vi "ROI_to_Size.vi"(11 "Actual ROI":T1 {"Rotation" format="%.2f"; "Left" scale=0.0..1024.0; "Right" scale=0.0..1024.0}) -> (3 "Image Size":cluster{"X":i32, "Y":i32})   [LabVIEW 2014]
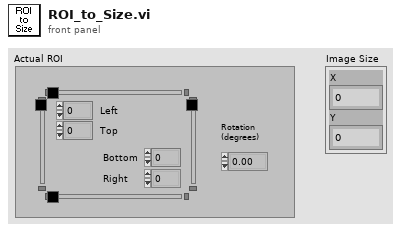
[diagram p1: front panel]
types:
  T1 = typedef "IMAQ Rectangle" = cluster{"Left":i32, "Top":i32, "Right":i32, "Bottom":i32, "Rotation":dbl}
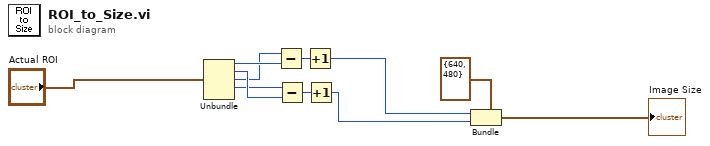
[diagram p0: block diagram]
diagram:
  n1 = Unbundle("Actual ROI") -> ("Left"=w3:i32, "Top"=w7:i32, "Right"=w2:i32, "Bottom"=w6:i32)  [unwired: 1 out]
  n2 = Subtract(x=w2, y=w3) -> (x-y=w4:i32)
  n3 = Subtract(x=w6, y=w7) -> (x-y=w5:i32)
  n4 = Increment(x=w4) -> (x+1=w9:i32)
  n5 = Increment(x=w5) -> (x+1=w10:i32)
  n6 = Bundle(cluster=cluster{"X":i32, "Y":i32} {"X"=640, "Y"=480} ("Image Size"), "X"=w9, "Y"=w10) -> (→"Image Size":cluster{"X":i32, "Y":i32})
